vi "12_FileWriter_FileReader.vi"(8 "error in (no error)":errorcluster) -> (0 "error out":errorcluster)   [LabVIEW 2014]
uses:
  SwabianInstruments.TimeTagger
panel:
  out "EventType":T1(array[ring])
  out "Channel":i32[](array[numeric])
  out "Timestamp":i64[](array[numeric])
  out "File path":path
  # "This example shows how to use FileWriter and FileReader for writing and reading\nthe time tag stream onto a disk.\n\nStep 1: \nThe FileWriter is used to dump the timetags from internal test signal into the filesystem.\n\nStep 2: \nThe FileReader is used to read the dumped timetags and display their values.\n\nStep 3:\nCleanup the temporary files"
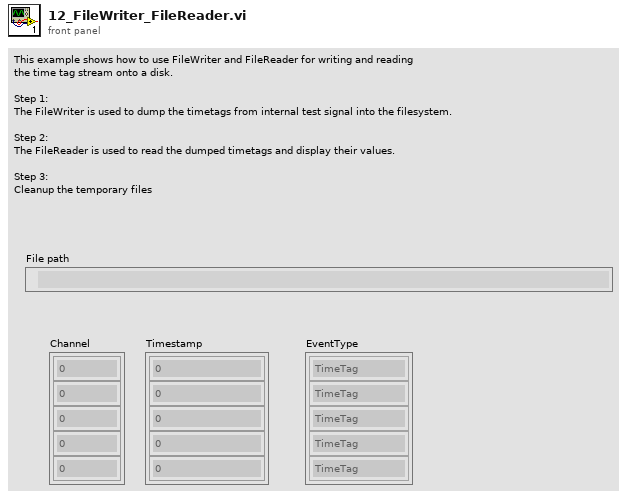
[diagram p1: front panel]
types:
  T1 = enum16{"TimeTag", "Error", "OverflowBegin", "OverflowEnd", "MissedEvents"}[]
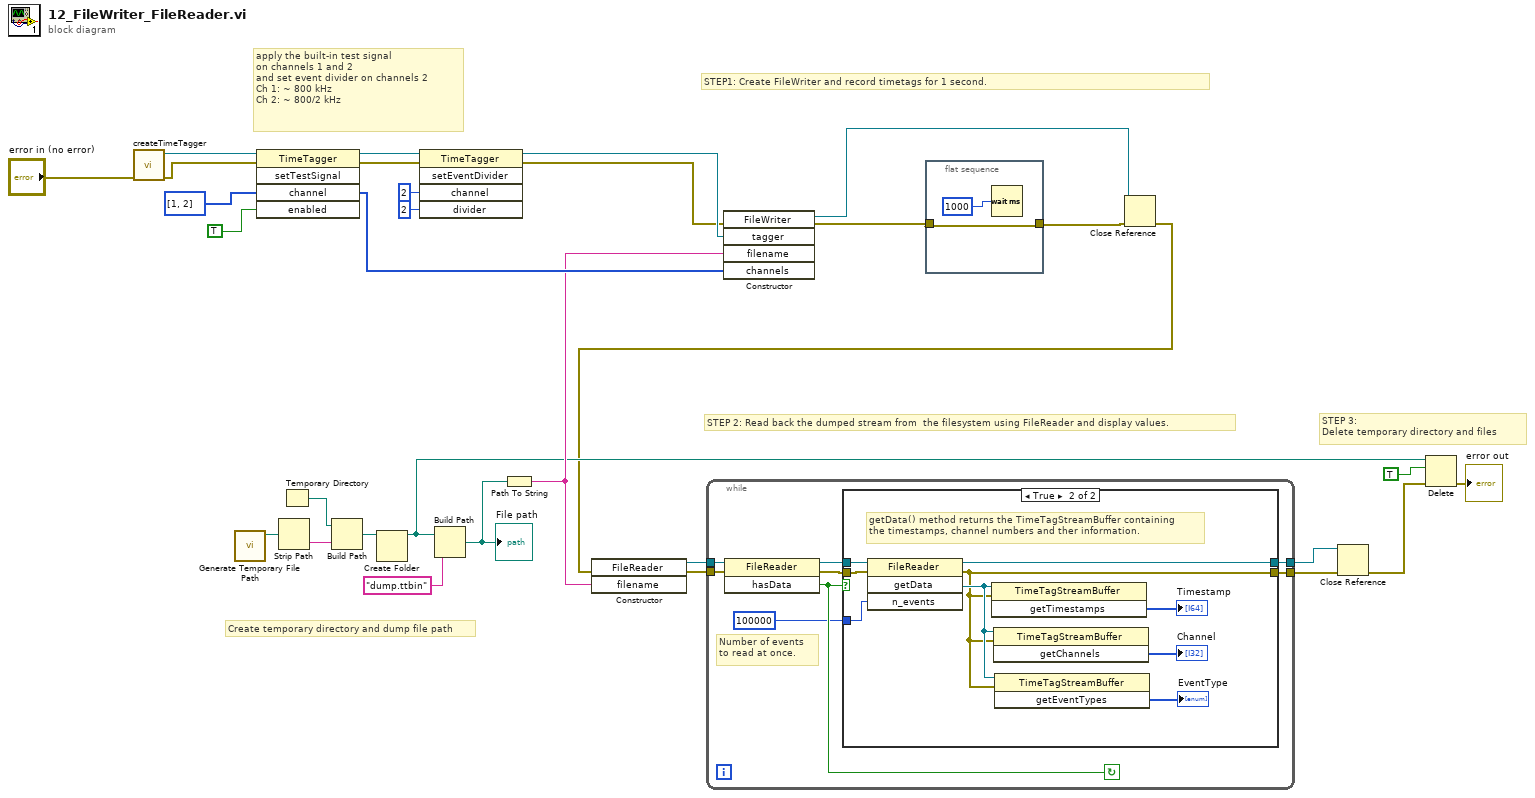
[diagram p0: block diagram]
diagram:
  # "STEP 3:\nDelete temporary directory and files"
  # "STEP 2: Read back the dumped stream from  the filesystem using FileReader and display values."
  # "STEP1: Create FileWriter and record timetags for 1 second."
  # "Create temporary directory and dump file path"
  # "apply the built-in test signal\non channels 1 and 2\nand set event divider on channels 2\nCh 1: ~ 800 kHz\nCh 2: ~ 800/2 kHz"
  n1 = call "createTimeTagger.vi"("error in (no error)"="error in (no error)") -> ("error out"=w26:errorcluster, "TimeTagger ref out"=w27:refnum<k24>)  [unwired: 9 in]
  n2 = call <vilib>:"Generate Temporary File Path.vi"() -> ("Unique Temporary File Path"=w22:path)  [unwired: 10 in, 1 out]
  n3 = invoke class="TimeTagger" method="setTestSignal"(reference=w27, error in=w26, "channel"=i32[] [1, 2], "enabled"=TRUE) -> (reference out=w29:refnum<k24>, error out=w28:errorcluster, "channel"=w18:i32[])  [unwired: 1 in, 2 out]
  n4 = Strip Path(path=w22) -> (name=w21:string)  [unwired: 1 out]
  n5 = Temporary Directory() -> (w20:path)
  n6 = Build Path(base path=w20, name or relative path=w21) -> (appended path=w13:path)
  n7 = Create Folder(path (use dialog)=w13) -> (created path=w12:path)  [unwired: 2 in, 2 out]
  n8 = invoke class="TimeTagger" method="setEventDivider"(reference=w29, error in=w28, "channel"=2, "divider"=u32 2) -> (reference out=w11:refnum<k24>, error out=w10:errorcluster)  [unwired: 1 in, 3 out]
  n9 = Build Path(base path=w12, name or relative path="dump.ttbin") -> (appended path=w19:path)
  "File path" <- w19
  n10 = Path To String(path=w19) -> (string=w17:string)
  n11 = constructor class="FileWriter"(error in=w10, "tagger"=w11, "filename"=w17, "channels"=w18) -> (reference out=w8:refnum<k24>, error out=w7:errorcluster)  [unwired: 2 in, 4 out]
  n12 = flat-sequence {
    tunnel: w7 -> [w32]
    tunnel: [w32] -> w6
    frame #0 {
      n13 = Wait (ms)(milliseconds to wait=u32 1000) -> ()  [unwired: 1 out]
    }
  }
  n14 = Close Reference(reference=w8, error in (no error)=w6) -> (error out=w9:errorcluster)
  n15 = constructor class="FileReader"(error in=w9, "filename"=w17) -> (reference out=w16:refnum<k24>, error out=w15:errorcluster)  [unwired: 2 in, 2 out]
  n16 = while {
    tunnel: w16 -> [w41]
    tunnel: w15 -> [w40]
    tunnel: [w35] -> w2
    tunnel: [w34] -> w3
    stop <- w39 continue-if-true
    # "Number of events \nto read at once."
    n17 = invoke class="FileReader" method="hasData"(reference=w41, error in=w40) -> (reference out=w38:refnum<k24>, error out=w37:errorcluster, "hasData"=w39:bool)  [unwired: 1 in]
    n18 = case shown="True" w39 {
      tunnel: w38 -> [w43 w52]
      tunnel: w37 -> [w42 w51]
      tunnel: u64 100000 ("n_events") -> [_ w50]
      tunnel: [w43 w45] -> w35
      tunnel: [w42 w44] -> w34
      frame False {
        # "No (more) data to read"
      }
      frame True {
        # "getData() method returns the TimeTagStreamBuffer containing \nthe timestamps, channel numbers and ther information."
        n19 = invoke class="FileReader" method="getData"(reference=w52, error in=w51, "n_events"=w50) -> (reference out=w45:refnum<k24>, error out=w44:errorcluster, "getData"=w49:refnum<k24>)  [unwired: 1 in, 1 out]
        n20 = invoke class="TimeTagStreamBuffer" method="getTimestamps"(reference=w49, error in=w44) -> ("getTimestamps"=→"Timestamp":i64[])  [unwired: 1 in, 2 out]
        n21 = invoke class="TimeTagStreamBuffer" method="getChannels"(reference=w49, error in=w44) -> ("getChannels"=→"Channel":i32[])  [unwired: 1 in, 2 out]
        n22 = invoke class="TimeTagStreamBuffer" method="getEventTypes"(reference=w49, error in=w44) -> ("getEventTypes"=→"EventType":u8[])  [unwired: 1 in, 2 out]
      }
    }
  }
  n23 = Close Reference(reference=w2, error in (no error)=w3) -> (error out=w1:errorcluster)
  n24 = Delete(path (use dialog)=w12, entire hierarchy (F)=TRUE, error in=w1) -> (error out=→"error out":errorcluster)  [unwired: 2 in, 2 out]
